vi "Overexposure Code.vi"() -> ()   [LabVIEW 2017]
uses:
  <vilib>/vision/NI_Vision_Development_Module.lvlib
panel:
  in  "Color Box":u32(colorbox)=16746240
  out "Image 3":T1(plugin-control)
  in  "Replace Value":sgl=1.0 format="%.2f"
  in  "selected path":path
  out "Image 2":T1(plugin-control)
  out "Image":T1(plugin-control)
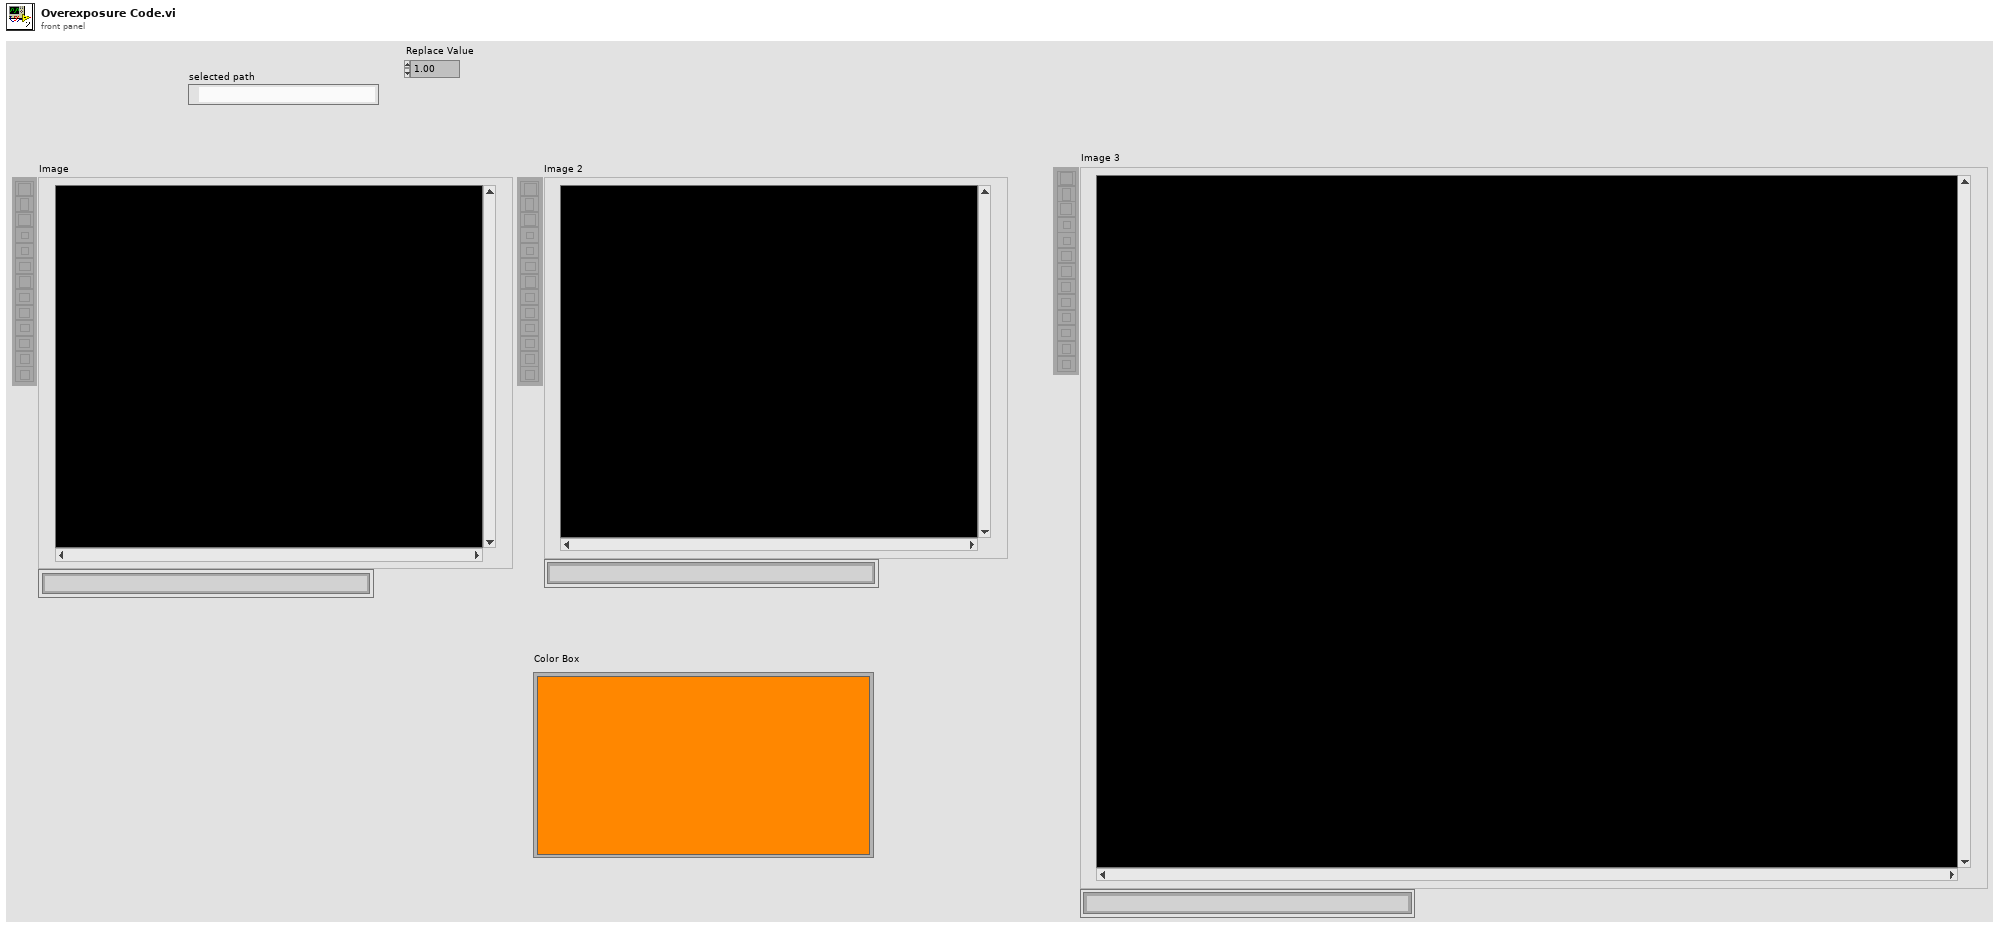
[diagram p1: front panel]
types:
  T1 = typedef "IMAQ Image.ctl" = refnum<image>
  T2 = typedef "Image Type" = u32
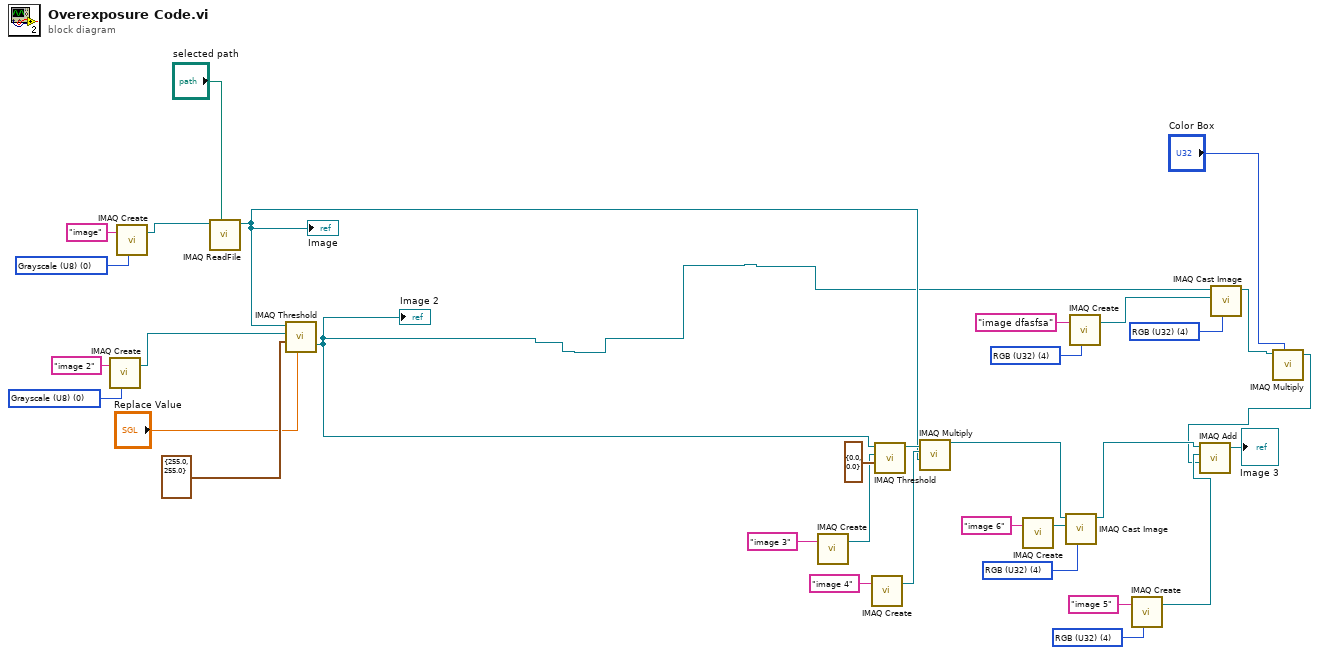
[diagram p0: block diagram]
diagram:
  w7 = T2 4 items=["Grayscale (U8)", "Grayscale (I16)", "Grayscale (SGL)", "Complex (CSG)", "RGB (U32)", "HSL (U32)", "RGB (U64)", "Grayscale (U16)"] ("Image Type")
  w12 = T2 4 items=["Grayscale (U8)", "Grayscale (I16)", "Grayscale (SGL)", "Complex (CSG)", "RGB (U32)", "HSL (U32)", "RGB (U64)", "Grayscale (U16)"] ("Image Type")
  w13 = T2 4 items=["Grayscale (U8)", "Grayscale (I16)", "Grayscale (SGL)", "Complex (CSG)", "RGB (U32)", "HSL (U32)", "RGB (U64)", "Grayscale (U16)"] ("Image Type")
  w15 = T2 4 items=["Grayscale (U8)", "Grayscale (I16)", "Grayscale (SGL)", "Complex (CSG)", "RGB (U32)", "HSL (U32)", "RGB (U64)", "Grayscale (U16)"] ("Image Type")
  w29 = T2 0 items=["Grayscale (U8)", "Grayscale (I16)", "Grayscale (SGL)", "Complex (CSG)", "RGB (U32)", "HSL (U32)", "RGB (U64)", "Grayscale (U16)"] ("Image Type")
  w30 = T2 0 items=["Grayscale (U8)", "Grayscale (I16)", "Grayscale (SGL)", "Complex (CSG)", "RGB (U32)", "HSL (U32)", "RGB (U64)", "Grayscale (U16)"] ("Image Type")
  n1 = call "IMAQ Create"("Image Name"="image 2", "Image Type"=w29) -> ("New Image"=w27:T1)  [unwired: 3 in, 1 out]
  n2 = call "IMAQ Create"("Image Name"="image", "Image Type"=w30) -> ("New Image"=w32:T1)  [unwired: 3 in, 1 out]
  n3 = call "IMAQ ReadFile"("File Path"="selected path", "Image"=w32) -> ("Image Out"=w16:T1)  [unwired: 5 in, 4 out]
  "Image" <- w16
  n4 = call "IMAQ Threshold"("Replace Value"="Replace Value", "Range"=cluster{"Lower value":sgl, "Upper value":sgl} {"Lower value"=255.0, "Upper value"=255.0}, "Image Dst"=w27, "Image Src"=w16) -> ("Image Dst Out"=w1:T1)  [unwired: 6 in, 1 out]
  "Image 2" <- w1
  n5 = call "IMAQ Create"("Image Name"="image 3") -> ("New Image"=w22:T1)  [unwired: 4 in, 1 out]
  n6 = call "IMAQ Create"("Image Name"="image 4") -> ("New Image"=w20:T1)  [unwired: 4 in, 1 out]
  n7 = call "IMAQ Threshold"("Range"=cluster{"Lower value":sgl, "Upper value":sgl} {"Lower value"=0.0, "Upper value"=0.0}, "Image Dst"=w22, "Image Src"=w1) -> ("Image Dst Out"=w19:T1)  [unwired: 7 in, 1 out]
  n8 = call "IMAQ Multiply"("Image Src A"=w19, "Image Dst"=w20, "Image Src B"=w16) -> ("Image Dst Out"=w6:T1)  [unwired: 4 in, 1 out]
  n9 = call "IMAQ Create"("Image Name"="image 6") -> ("New Image"=w8:T1)  [unwired: 4 in, 1 out]
  n10 = call "IMAQ Cast Image"("Image Type"=w7, "Image Dst"=w8, "Image Src"=w6) -> ("Image Dst Out"=w5:T1)  [unwired: 7 in, 1 out]
  n11 = call "IMAQ Create"("Image Name"="image dfasfsa", "Image Type"=w12) -> ("New Image"=w11:T1)  [unwired: 3 in, 1 out]
  n12 = call "IMAQ Create"("Image Name"="image 5", "Image Type"=w15) -> ("New Image"=w14:T1)  [unwired: 3 in, 1 out]
  n13 = call "IMAQ Cast Image"("Image Type"=w13, "Image Dst"=w11, "Image Src"=w1) -> ("Image Dst Out"=w4:T1)  [unwired: 7 in, 1 out]
  n14 = call "IMAQ Multiply"("Image Src A"=w4, "Constant"="Color Box") -> ("Image Dst Out"=w3:T1)  [unwired: 5 in, 1 out]
  n15 = call "IMAQ Add"("Image Src A"=w5, "Image Dst"=w14, "Image Src B"=w3) -> ("Image Dst Out"=→"Image 3":T1)  [unwired: 4 in, 1 out]
